vi "Get XY4 Params.vi"(11 "XY-4 Parameters":T1={"Path to CPMG Burner"=path "C:/Users/Loncar/Desktop/ESR VIs - Srujan/Sam Kim/PB/SpinEchoBurn.exe", "Window 1 time (s)"=3e-06, "Window 1 active channels"=[FALSE, FALSE, FALSE, TRUE], "Window 10 time (s)"=3e-06, "Window 10 active channels"=[FALSE, FALSE, FALSE, TRUE], "Window 2 time (s)"=0.0, "Window 2 active channels"=[], "Window 4 min time (s) "=0.0, "Window 4 active channels"=[FALSE], "Window 8 time (s)"=7.5e-07, "Window 8 active channels"=[FALSE, FALSE, FALSE, TRUE], "Window 9 time (s)"=2e-07, "Window 9 active channels "=[FALSE, FALSE, TRUE, TRUE], "# time points"=1, "Window 11 time (s)"=0.0, "Window 11 active channels"=[FALSE, FALSE, TRUE, TRUE], "Window 12 time (s)"=1e-07, "Window 12 active channels"=[], "Window 4 max time (s)"=0.0, "Window 3 time (s)"=0.0, "Window 5 time (s)"=5e-06, "Window 3 active channels"=[TRUE, FALSE, FALSE, FALSE], "Window 5c active channels"=[TRUE, FALSE, FALSE, FALSE], "# pulse sequences"=1, "# samples before track"=0, "Window 5a active channels"=[TRUE, FALSE, FALSE, FALSE]} {"# pulse sequences" min=1; "# time points" min=2}) -> (0 "max time":dbl, 1 "min time":dbl, 2 "# time points":i32, 3 "# samples":i32, 4 "String":string)   [LabVIEW 2012]
uses:
  Window Parameters-XY4.ctl
panel:
  # "pulse=XYXY"
  # "max: ~350"
  # "x 4=#pi pulses"
  # "Green AOM"
  # "Initialization"
  # "All off"
  # "Wait"
  # "MW pulse 1\n(pi/2)"
  # "MW"
  # "Free precession\n(T/2)"
  # "All off"
  # "MW (X)"
  # "MW pulse 2\n(pi)"
  # "MW90 (Y)"
  # "Pulse Sequence=[T/2-Pi-T-Pi90-T-Pi-T-Pi90-T/2]^N\nMW pulse 1 (pi/2)"
  # "Window 4-5a-g-6\nWindow 7"
  # "Green AOM"
  # "Wait for green"
  # "Green AOM,\ncounter sample clk"
  # "Readout"
  # "Green AOM"
  # "Repump"
  # "Green AOM,\ncounter sample clk"
  # "Reference"
  # "Wait (nominal)"
  # "All off"
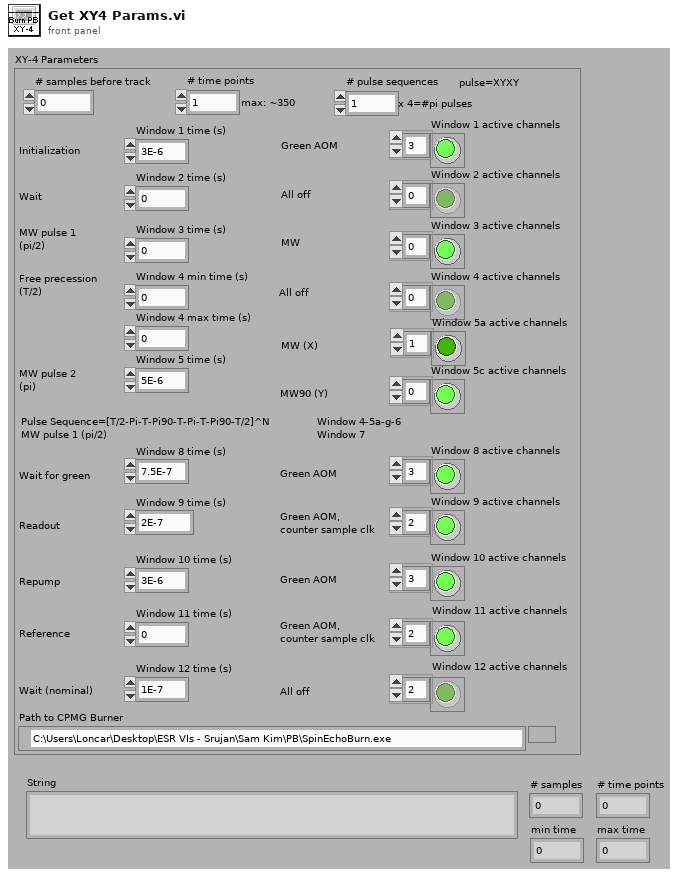
[diagram p1: front panel]
types:
  T1 = typedef "Window Parameters-XY4.ctl" = cluster{"Path to CPMG Burner":path, "Window 1 time (s)":dbl, "Window 1 active channels":bool[], "Window 10 time (s)":dbl, "Window 10 active channels":bool[], "Window 2 time (s)":dbl, "Window 2 active channels":bool[], "Window 4 min time (s) ":dbl, "Window 4 active channels":bool[], "Window 8 time (s)":dbl, "Window 8 active channels":bool[], "Window 9 time (s)":dbl, "Window 9 active channels ":bool[], "# time points":i32, "Window 11 time (s)":dbl, "Window 11 active channels":bool[], "Window 12 time (s)":dbl, "Window 12 active channels":bool[], "Window 4 max time (s)":dbl, "Window 3 time (s)":dbl, "Window 5 time (s)":dbl, "Window 3 active channels":bool[], "Window 5c active channels":bool[], "# pulse sequences":i32, "# samples before track":i32, "Window 5a active channels":bool[]}
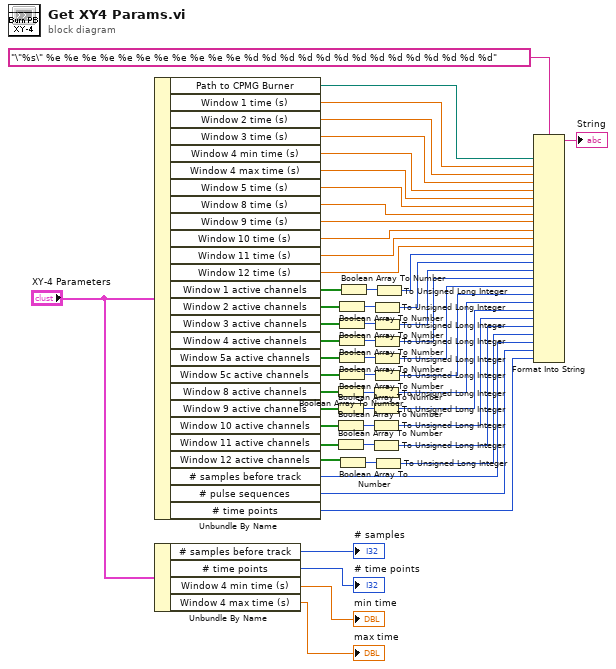
[diagram p0: block diagram]
diagram:
  n1 = Unbundle By Name("XY-4 Parameters") -> ("Path to CPMG Burner"=w44:path, "Window 1 time (s)"=w48:dbl, "Window 2 time (s)"=w47:dbl, "Window 3 time (s)"=w46:dbl, "Window 4 min time (s)"=w45:dbl, "Window 4 max time (s)"=w43:dbl, "Window 5 time (s)"=w42:dbl, "Window 8 time (s)"=w41:dbl, "Window 9 time (s)"=w11:dbl, "Window 10 time (s)"=w30:dbl, "Window 11 time (s)"=w29:dbl, "Window 12 time (s)"=w28:dbl, "Window 1 active channels"=w19:bool[], "Window 2 active channels"=w18:bool[], "Window 3 active channels"=w17:bool[], "Window 4 active channels"=w36:bool[], "Window 5a active channels"=w27:bool[], "Window 8 active channels"=w26:bool[], "Window 9 active channels"=w25:bool[], "Window 12 active channels"=w7:bool[], "# samples before track"=w14:i32, "# pulse sequences"=w13:i32, "# time points"=w12:i32)  [unwired: 3 out]
  n2 = Unbundle By Name("XY-4 Parameters") -> ("# samples before track"=→"# samples":i32, "# time points"=→"# time points":i32, "Window 4 min time (s)"=→"min time":dbl, "Window 4 max time (s)"=→"max time":dbl)
  n3 = Boolean Array To Number(Boolean array=w27) -> (number=w51:u32)
  n4 = Boolean Array To Number(Boolean array=w26) -> (number=w50:u32)
  n5 = Boolean Array To Number(Boolean array=w25) -> (number=w49:u32)
  n6 = Boolean Array To Number(Boolean array=w7) -> (number=w9:u32)
  n7 = Boolean Array To Number(Boolean array=w17) -> (number=w20:u32)
  n8 = Boolean Array To Number(Boolean array=w19) -> (number=w40:u32)
  n9 = Boolean Array To Number(Boolean array=w18) -> (number=w39:u32)
  n10 = Boolean Array To Number(Boolean array=w17) -> (number=w38:u32)
  n11 = Boolean Array To Number(Boolean array=w36) -> (number=w37:u32)
  n12 = Boolean Array To Number(Boolean array=w7) -> (number=w8:u32)
  n13 = Boolean Array To Number(Boolean array=w18) -> (number=w21:u32)
  n14 = To Unsigned Long Integer(number=w51) -> (unsigned 32bit integer=w24:u32)
  n15 = To Unsigned Long Integer(number=w50) -> (unsigned 32bit integer=w23:u32)
  n16 = To Unsigned Long Integer(number=w49) -> (unsigned 32bit integer=w22:u32)
  n17 = To Unsigned Long Integer(number=w9) -> (unsigned 32bit integer=w10:u32)
  n18 = To Unsigned Long Integer(number=w20) -> (unsigned 32bit integer=w15:u32)
  n19 = To Unsigned Long Integer(number=w40) -> (unsigned 32bit integer=w35:u32)
  n20 = To Unsigned Long Integer(number=w39) -> (unsigned 32bit integer=w34:u32)
  n21 = To Unsigned Long Integer(number=w38) -> (unsigned 32bit integer=w33:u32)
  n22 = To Unsigned Long Integer(number=w37) -> (unsigned 32bit integer=w32:u32)
  n23 = To Unsigned Long Integer(number=w8) -> (unsigned 32bit integer=w6:u32)
  n24 = To Unsigned Long Integer(number=w21) -> (unsigned 32bit integer=w16:u32)
  n25 = Format Into String(format string="\"%s\" %e %e %e %e %e %e %e %e %e %e %e %d %d %d %d %d %d %d %d %d %d %d %d %d %d", w44, w48, w47, w46, w45, w43, w42, w41, w11, w30, w29, w28, w16, w15, w35, w34, w33, w32, w24, w23, w22, w10, w6, w14, w13, w12) -> (resulting string=→"String":string)  [unwired: 2 in, 1 out]
